vi "Write cyclical pattern.vi"(8 "error in (no error)":errorcluster, 10 "cyclical pattern":T1, 11 "Device in":refnum<class "Device.lvclass">) -> (0 "error out":errorcluster, 3 "Device out":refnum<class "Device.lvclass">)   [LabVIEW 2023, in "Device.lvlib" / "Device.lvclass"]
uses:
  Device.lvclass
  Device.lvclass/Device.ctl
  Control/cyclical pattern.ctl
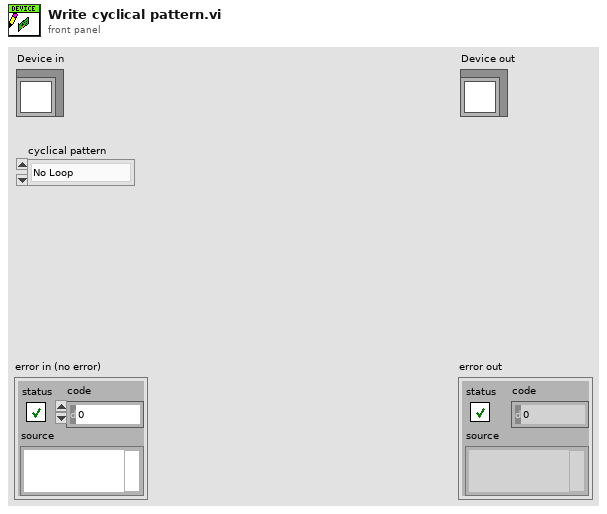
[diagram p1: front panel]
types:
  T1 = typedef "Device.lvlib/Device.lvclass/cyclical pattern.ctl" = enum16{"No Loop", "Fastest", "Timer"}
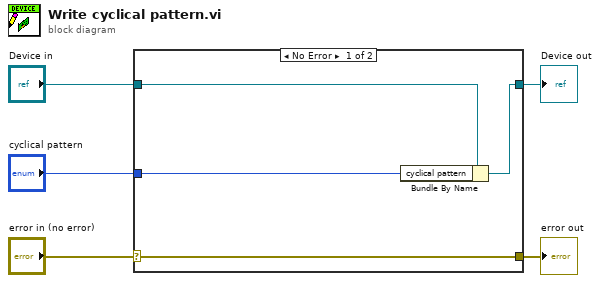
[diagram p0: block diagram]
diagram:
  n1 = case shown="No Error" "error in (no error)" {
    selector: "error in (no error)" -> [w9 w10]
    tunnel: [w9 w10] -> w4
    tunnel: [w7 w11] -> w2
    tunnel: "Device in" -> [w8 w11]
    tunnel: "cyclical pattern" -> [w6 _]
    frame No Error {
      n2 = Bundle By Name(cluster=w8, "cyclical pattern"=w6) -> (w7:refnum<class "Device.lvclass">)
    }
    frame Error {
    }
  }
  "error out" <- w4
  "Device out" <- w2
